vi "Memory Game trial.vi"   [LabVIEW 2019]
uses:
  <vilib>/numeric/Random Number (Range) U64.vi
  <vilib>/numeric/sub_Random U32.vi
panel:
  # "Memory Mobile Game"
  # "Dial the number shown in the display"
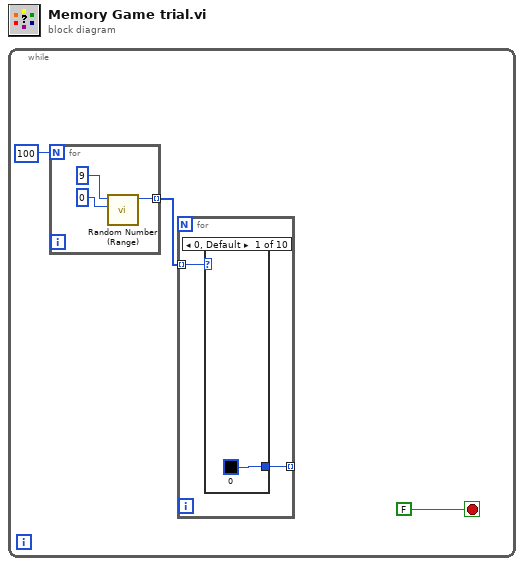
[diagram p0: block diagram]
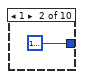
[diagram p2: hidden frame]
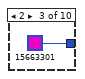
[diagram p3: hidden frame]
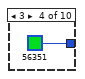
[diagram p4: hidden frame]
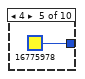
[diagram p5: hidden frame]
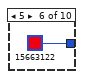
[diagram p6: hidden frame]
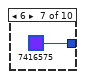
[diagram p7: hidden frame]
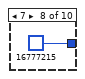
[diagram p8: hidden frame]
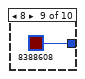
[diagram p9: hidden frame]
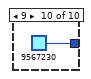
[diagram p10: hidden frame]
diagram:
  n1 = while {
    stop <- FALSE stop-if-true
    # "Main loop, run  once per game"
    n2 = for {
      N: 100 -> [_]
      tunnel: [w16] -> w1 mode=indexing
      # "generate randome sequence of\ncolor indices (0 .. 9)"
      n3 = call-poly <vilib>:"Random Number (Range).vi"("lower bound (0)"=u64 0, "upper bound (100)"=u64 9) -> ("number"=w16:u64)  [unwired: 9 in]
    }
    n4 = for {
      tunnel: w1 -> [w5] mode=indexing
      tunnel: [w4] -> _ mode=indexing
      # "generate sequence of colors"
      n5 = case shown="0, Default" w5 {
        tunnel: [u32 0 ("Color Box") u32 16777224 ("Color Box") u32 15663301 ("Color Box") u32 56351 ("Color Box") u32 16775978 ("Color Box") u32 15663122 ("Color Box") u32 7416575 ("Color Box") u32 16777215 ("Color Box") u32 8388608 ("Color Box") u32 9567230 ("Color Box")] -> w4
        frame 0, Default {
        }
        frame 1 {
        }
        frame 2 {
        }
        frame 3 {
        }
        frame 4 {
        }
        frame 5 {
        }
        frame 6 {
        }
        frame 7 {
        }
        frame 8 {
        }
        frame 9 {
        }
      }
    }
  }
